vi "front pannel position and size.vi"(8 "error in":errorcluster, 10 "Position":T1) -> (0 "error out":errorcluster)   [LabVIEW 2020]
uses:
  <vilib>/Utility/miscctls.llb/LVPositionTypeDef.ctl
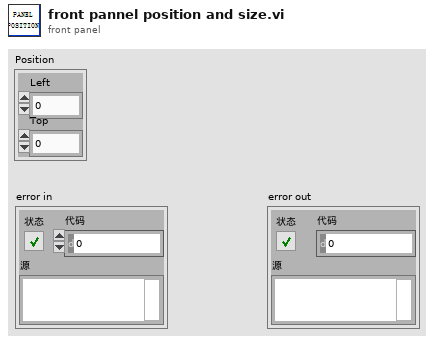
[diagram p1: front panel]
types:
  T1 = typedef "LVPositionTypeDef.ctl" = cluster{"Left":i32, "Top":i32}
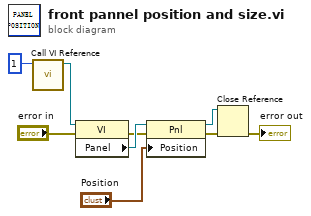
[diagram p0: block diagram]
diagram:
  n1 = call "Call VI Reference.vi"("last level"=1 ("上层调用索引")) -> ("vi reference out"=w8:refnum<vi>)  [unwired: 9 in, 1 out]
  n2 = property class="VI"(reference=w8, error in="error in") -> (error out=w5:errorcluster, "Panel"=w7:refnum<vi>)  [unwired: 1 out]
  n3 = property class="Pnl"(reference=w7, error in=w5, "Position"="Position") -> (reference out=w3:refnum<vi>, error out=w4:errorcluster)
  n4 = Close Reference(reference=w3, error in (no error)=w4) -> (error out=→"error out":errorcluster)
